vi "Add Remove Test.vi"() -> ()   [LabVIEW 2014, in "FPGA Windows Tests.lvlib"]
doc: "Tests the Add Line and Remove Line functions."
uses:
  FPGA Windows Tests.lvlib
  module/configuration/FPGA Module configuration.lvclass
  <vilib>/NI/Tag Bus/tag/Data Type.ctl
  <vilib>/NI/Tag Bus/tag/tag descriptor.lvclass
  module/configuration/Line.ctl
  fpga channel/FPGA Channel.lvclass
  <vilib>/NI/Tag Bus Module Framework/channel/channel classification.ctl
  <vilib>/NI/Tag Bus Module Framework/channel/TBM channel.lvclass
panel:
  out "Deleted Line":string
  out "Success Delete":bool
  out "error out":errorcluster
  out "Success ADD":bool
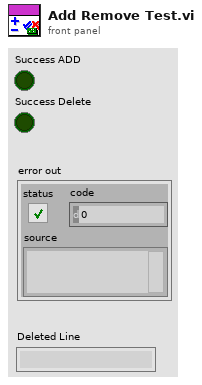
[diagram p1: front panel]
types:
  T1 = typedef "TBM channel.lvclass/channel classification.ctl" = enum16{"input data", "output data", "processing parameter", "processing result"}
  T2 = typedef "FPGA Module configuration.lvclass/Line.ctl" = cluster{"Channel":refnum<class "FPGA Channel.lvclass">}
  T3 = typedef "tag bus.lvlib/tag descriptor.lvclass/Data Type.ctl" = enum16{"Double", "Single", "I64", "I32", "I16", "I8", "U64", "U32", "U16", "U8", "Boolean", "String", "Array of Double", "Array of Single", "Array of I64", "Array of I32", "Array of I16", "Array of I8", "Array of U64", "Array of U32", "Array of U16", "Array of U8", "Array of Boolean", "Array of String"}
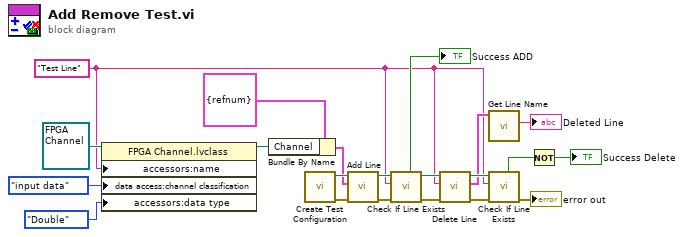
[diagram p0: block diagram]
diagram:
  w1 = "Test Line" ("channel name")
  n1 = property class="FPGA Channel.lvclass"(reference=refnum<class "FPGA Channel.lvclass"> refnum ("Channel"), "accessors:name"=w1, "data access:channel classification"=channel_classification."input data" ("channel classification"), "accessors:data type"=Data_Type."Double" ("data type")) -> (reference out=w5:refnum<class "FPGA Channel.lvclass">)  [unwired: 1 in, 1 out]
  n2 = Bundle By Name(cluster=T2 {"Channel"=refnum} ("Line"), "Channel"=w5) -> (w19:T2)
  n3 = call "Create Test Configuration.vi"() -> ("error out"=w13:errorcluster, "Module Configuration"=w21:refnum<class "FPGA Module configuration.lvclass">)  [unwired: 6 in, 4 out]
  n4 = call "Add Line.vi"("error in"=w13, "Line"=w19, "FPGA Module configuration in"=w21) -> ("error out"=w15:errorcluster, "FPGA Module configuration out"=w18:refnum<class "FPGA Module configuration.lvclass">)  [unwired: 6 in, 1 out]
  n5 = call-dynamic "Check If Line Exists.vi"("error in"=w15, "Name to Locate"=w1, "FPGA Module configuration in"=w18) -> ("error out"=w14:errorcluster, "FPGA Module configuration out"=w17:refnum<class "FPGA Module configuration.lvclass">, "Found?"=→"Success ADD":bool)  [unwired: 4 in, 2 out]
  n6 = call "Delete Line.vi"("error in"=w14, "Line Name"=w1, "FPGA Module configuration in"=w17) -> ("error out"=w12:errorcluster, "Deleted Line"=w7:T2, "FPGA Module configuration out"=w10:refnum<class "FPGA Module configuration.lvclass">)  [unwired: 6 in]
  n7 = call "Get Line Name.vi"("Line in"=w7) -> ("Name"=→"Deleted Line":string)  [unwired: 8 in, 2 out]
  n8 = call-dynamic "Check If Line Exists.vi"("error in"=w12, "Name to Locate"=w1, "FPGA Module configuration in"=w10) -> ("error out"=→"error out":errorcluster, "Found?"=w9:bool)  [unwired: 4 in, 3 out]
  n9 = Not(x=w9) -> (.not. x?=→"Success Delete":bool)
